vi "DriveForwardRTv2.vi"   [LabVIEW 2015]
uses:
  ShiftGlobals.vi
  MotorPositionGlobals.vi
  navx-mxp/labview/navX Library v2/navX Library v2.lvlib
types:
  T1 = typedef "WPI_MotorControlDeviceRef.ctl" = cluster{"DeviceStatus":errorcluster, "Type":T2, "PWM":cluster{"PWM Channel":T3, "DeadBand":T4}, "CAN":cluster{"Device Number":u8, "Control Mode":T5, "Semaphore":T6, "Max Vout":dbl, "TalonSRX Control Mode":T7}, "Invert":bool}
  T2 = typedef "WPI_MotorControlType.ctl" = enum16{"PWM", "CAN", "CANTalonSRX"}
  T3 = typedef "FPGA_DIOPWMChannel.ctl" = enum8{"PWM 0", "PWM 1", "PWM 2", "PWM 3", "PWM 4", "PWM 5", "PWM 6", "PWM 7", "PWM 8", "PWM 9", "PWM MXP 0", "PWM MXP 1", "PWM MXP 2", "PWM MXP 3", "PWM MXP 4", "PWM MXP 5", "PWM MXP 6", "PWM MXP 7", "PWM MXP 8", "PWM MXP 9", "Invalid"}
  T4 = typedef "WPI_PWMDeadband.ctl" = cluster{"Name":string, "maxPositivePwm":i32, "minPositivePwm":i32, "centerPwm":i32, "maxNegativePwm":i32, "minNegativePwm":i32, "angularRange":u16}
  T5 = typedef "WPI_CANJaguar_ControlMode.ctl" = enum8{"Percent VBus", "Current", "Speed", "Position", "Voltage"}
  T6 = typedef "Semaphore RefNum" = refnum<k1>
  T7 = typedef "WPI_CANTalonSRX_APIControlMode.ctl" = enum8{"Percent VBus", "Speed", "Position", "Slave", "Unchanged / Invalid", "Voltage Compensation", "Current", "Motion Profile"}
  T8 = typedef "navX Library v2.lvlib/Z900_navX_DeviceTypeDef.ctl" = cluster{"Interface":cluster{"Protocol":T9, "Update Rate (4Hz-100Hz)":u8, "navX Open TypeDef":variant}, "Notify Packet":refnum<notifier>, "Loop VI Refnum":refnum<vi>, "Ready to Close Occurrence Refnum":refnum<k4>}
  T9 = typedef "navX Library v2.lvlib/Z900_navX_ProtocolTypeDef.ctl" = enum16{"SERIAL", "I2C", "SPI"}
  T10 = typedef "WPI_CANTalonSRX_GlobalStatus.ctl" = cluster{"Applied Throttle":dbl, "Module Enabled":bool, "CAN Error":errorcluster, "Closed Loop Error":dbl, "Forward Limit Switch Closed":bool, "Reverse Limit Switch Closed":bool, "Sensor Position":dbl, "Sensor Velocity":dbl, "Current":dbl, "Sticky Fault - Over Temp":bool, "Sticky Fault - Under Voltage":bool, "Sticky Fault - Forward Limit":bool, "Sticky Fault - Reverse Limit":bool, "Sticky Fault - Forward Soft Limit":bool, "Sticky Fault - Reverse Soft Limit":bool, "Brake is Enabled":bool, "Encoder Position":dbl, "Encoder Velocity":dbl, "Encoder Index Count":dbl, "Encoder A Pin State":bool, "Encoder B Pin State":bool, "Encoder Index Pin State":bool, "Analog In":dbl, "Analog In Velocity":dbl, "Temperature (C)":dbl, "Battery Voltage":dbl, "Control 5 Is Supported":bool, "Current Profile Slot Select":dbl, "Pos Div 8":bool, "Vel Div 4":bool, "Pulse Width Position":i32, "Pulse Width Velocity":i32, "Pulse Width Rise To Rise (us)":i32, "Pulse Width Rise To Fall (us)":i32, "Mot Prof Active Is Under Run":bool, "Mot Prof Active Has Under Run":bool, "Mot Prof Active Is Last":bool, "Mot Prof Active Velocity Only":bool, "Mot Prof Active Is Valid":bool, "Mot Prof Buffer Is Full":bool, "Mot Prof Active Profile Slot Select":i32, "Mot Prof NextID":i32, "Mot Prof Count":i32, "Mot Prof Active Velocity":dbl, "Mot Prof Active Position":dbl, "Mot Prof Output Enable":i32}
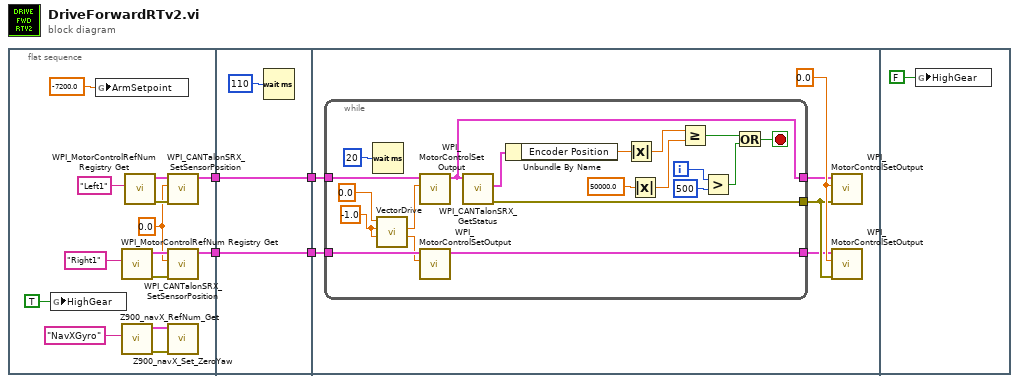
[diagram p0: block diagram]
diagram:
  n1 = flat-sequence {
    tunnel: [w11] -> w4
    tunnel: [w10] -> w3
    tunnel: w4 -> [w21]
    tunnel: [w21] -> w1
    tunnel: w3 -> [w20]
    tunnel: [w20] -> w2
    tunnel: w2 -> [w25]
    tunnel: w1 -> [w24]
    frame #0 {
      w12 = 0.0 ("New Sensor Position")
      n2 = global write "ShiftGlobals.vi" "HighGear"(TRUE ("HighGear")) -> ()
      n3 = global write "MotorPositionGlobals.vi" "ArmSetpoint"(-7200.0 ("ArmSetpoint")) -> ()
      n4 = call <vilib>:"WPI_MotorControlRefNum Registry Get.vi"("refnum name"="Right1") -> ("error out"=w16:errorcluster, "MotorControlDevRef"=w15:T1)  [unwired: 9 in]
      n5 = call "Z900_navX_RefNum_Get.vi"("refnum name"="NavXGyro") -> ("error out"=w6:errorcluster, "navX Device"=w7:T8)  [unwired: 9 in]
      n6 = call <vilib>:"WPI_MotorControlRefNum Registry Get.vi"("refnum name"="Left1") -> ("error out"=w14:errorcluster, "MotorControlDevRef"=w13:T1)  [unwired: 9 in]
      n7 = call <vilib>:"WPI_CANTalonSRX_SetSensorPosition.vi"("error in (no error)"=w14, "New Sensor Position"=w12, "CAN Talon SRX Ref"=w13) -> ("CAN Talon SRX Ref"=w10:T1)  [unwired: 7 in, 1 out]
      n8 = call <vilib>:"WPI_CANTalonSRX_SetSensorPosition.vi"("error in (no error)"=w16, "New Sensor Position"=w12, "CAN Talon SRX Ref"=w15) -> ("CAN Talon SRX Ref"=w11:T1)  [unwired: 7 in, 1 out]
      n9 = call "Z900_navX_Set_ZeroYaw.vi"("error in (no error)"=w6, "navX Device"=w7) -> ()  [unwired: 8 in, 2 out]
    }
    frame #1 {
      n10 = Wait (ms)(milliseconds to wait=u32 110) -> ()  [unwired: 1 out]
    }
    frame #2 {
      w27 = 0.0 ("Output")
      n11 = while {
        tunnel: [w36] -> w26
        tunnel: w25 -> [w35]
        tunnel: w24 -> [w34]
        tunnel: [w33] -> w23
        tunnel: [w32] -> w22
        i -> [w42]
        stop <- w44 stop-if-true
        w29 = -1.0 ("Output")
        n12 = Wait (ms)(milliseconds to wait=u32 20) -> ()  [unwired: 1 out]
        n13 = call "VectorDrive.vi"("RightMotorInput"=w29, "LeftMotorInput"=w29, "setpoint"=0.0) -> ("RightMotorOutput"=w30:dbl, "LeftMotorOutput"=w31:dbl)  [unwired: 7 in]
        n14 = call <vilib>:"WPI_MotorControlSetOutput.vi"("Output"=w31, "MotorControlDevRef"=w35) -> ("MotorControlDevRef"=w33:T1)  [unwired: 7 in, 2 out]
        n15 = call <vilib>:"WPI_MotorControlSetOutput.vi"("Output"=w30, "MotorControlDevRef"=w34) -> ("MotorControlDevRef"=w32:T1)  [unwired: 7 in, 2 out]
        n16 = call <vilib>:"WPI_CANTalonSRX_GetStatus.vi"("CAN Talon SRX Ref"=w33) -> ("error out"=w36:errorcluster, "Talon SRX Status"=w46:T10)  [unwired: 8 in, 1 out]
        n17 = Unbundle By Name(w46) -> ("Encoder Position"=w40:dbl)
        n18 = Absolute Value(x=w40) -> (abs(x)=w39:dbl)
        n19 = Absolute Value(x=50000.0) -> (abs(x)=w38:dbl)
        n20 = Greater Or Equal?(x=w39, y=w38) -> (x >= y?=w45:bool)
        n21 = Greater?(x=w42, y=500) -> (0:w43:bool)
        n22 = Or(x=w45, y=w43) -> (x .or. y?=w44:bool)
      }
      n23 = call <vilib>:"WPI_MotorControlSetOutput.vi"("error in (no error)"=w26, "Output"=w27, "MotorControlDevRef"=w23) -> ()  [unwired: 6 in, 3 out]
      n24 = call <vilib>:"WPI_MotorControlSetOutput.vi"("error in (no error)"=w26, "Output"=w27, "MotorControlDevRef"=w22) -> ()  [unwired: 6 in, 3 out]
    }
    frame #3 {
      n25 = global write "ShiftGlobals.vi" "HighGear"(FALSE ("HighGear")) -> ()
    }
  }
